vi "Custom SCP Command Page.vi"(8 "error in (no error)":errorcluster, 11 "Node Ptr":T1 format="%.0x") -> (0 "error out":errorcluster)   [LabVIEW 2023, in "Vires VTD System Explorer.lvlib"]
uses:
  Vires VTD System Explorer.lvlib
  <vilib>/NI VeriStand/Custom Device API/Custom Device Item Ref.ctl
  <vilib>/Utility/miscctls.llb/LVRowAndColumnTypeDef.ctl
  Shared/Constants.vi
  <vilib>/NI VeriStand/Custom Device API/Get Item Property (Boolean).vi
  <vilib>/NI VeriStand/Custom Device API/Set Item Property (Boolean).vi
  <vilib>/NI VeriStand/Custom Device API/Custom Device API.lvlib
  Shared/Vires VTD Shared.lvlib
panel:
  in  "Display hidden characters":bool
  in  "Default SCP Command ID":dbl
  in  "Command String":string
  in  "Down Arrow":bool
  in  "Up Arrow":bool
  in  "c SCP List":i32(listbox) caption="Custom SCP Commands List"
  in  "SHDocVw.IWebBrowser2":refnum<k7>(container)
  in  "Header":cluster{"Section Name":string}={"Section Name"="Custom Device Channel Settings"}
  in  "Description":string
  in  "Name":string
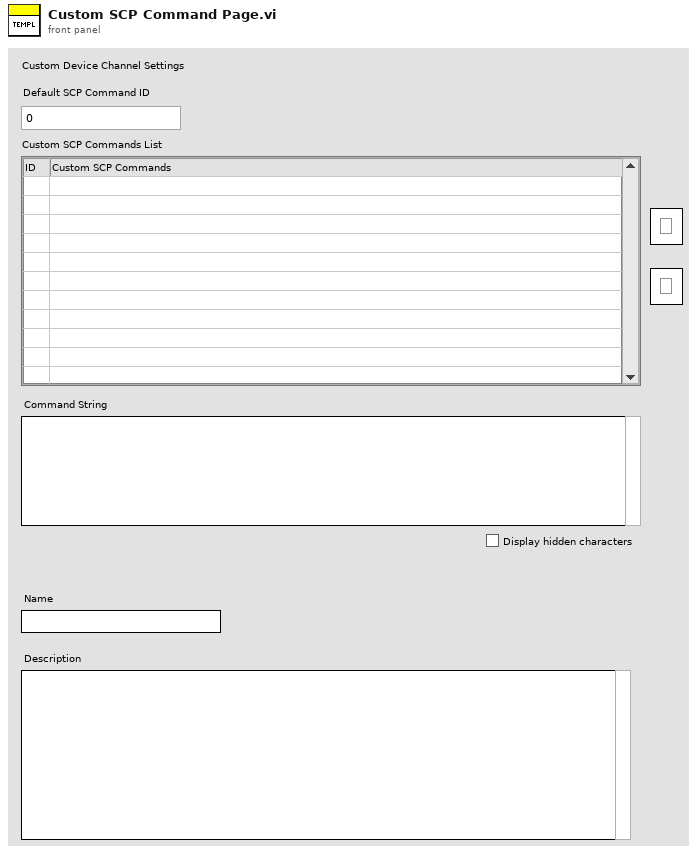
[diagram p1: front panel]
types:
  T1 = typedef "Custom Device API.lvlib/Custom Device Item Ref.ctl" = u64
  T2 = typedef "Custom Device API.lvlib/Custom Device Channel.ctl" = cluster{"Type":T3, "Units":string, "Default Value":dbl, "Faultable":bool, "Scalable":bool}
  T3 = typedef "Custom Device API.lvlib/Custom Device Channel Type.ctl" = enum16{"Input", "Output"}
  T4 = typedef "Custom Device API.lvlib/Custom Device Item Info.ctl" = cluster{"Name":string, "Is Channel":bool, "GUID":string, "Is Waveform":bool}
  T5 = typedef "LVRowAndColumnTypeDef.ctl" = cluster{"Row":i32, "Column":i32}
  T6 = typedef "Custom Device API.lvlib/Custom Device Commands.ctl" = enum16{"Default", "Item renamed", "Shutdown", "Dynamic button pressed"}
  T7 = typedef "LVPoint32TypeDef.ctl" = cluster{"Horizontal":i32, "Vertical":i32}
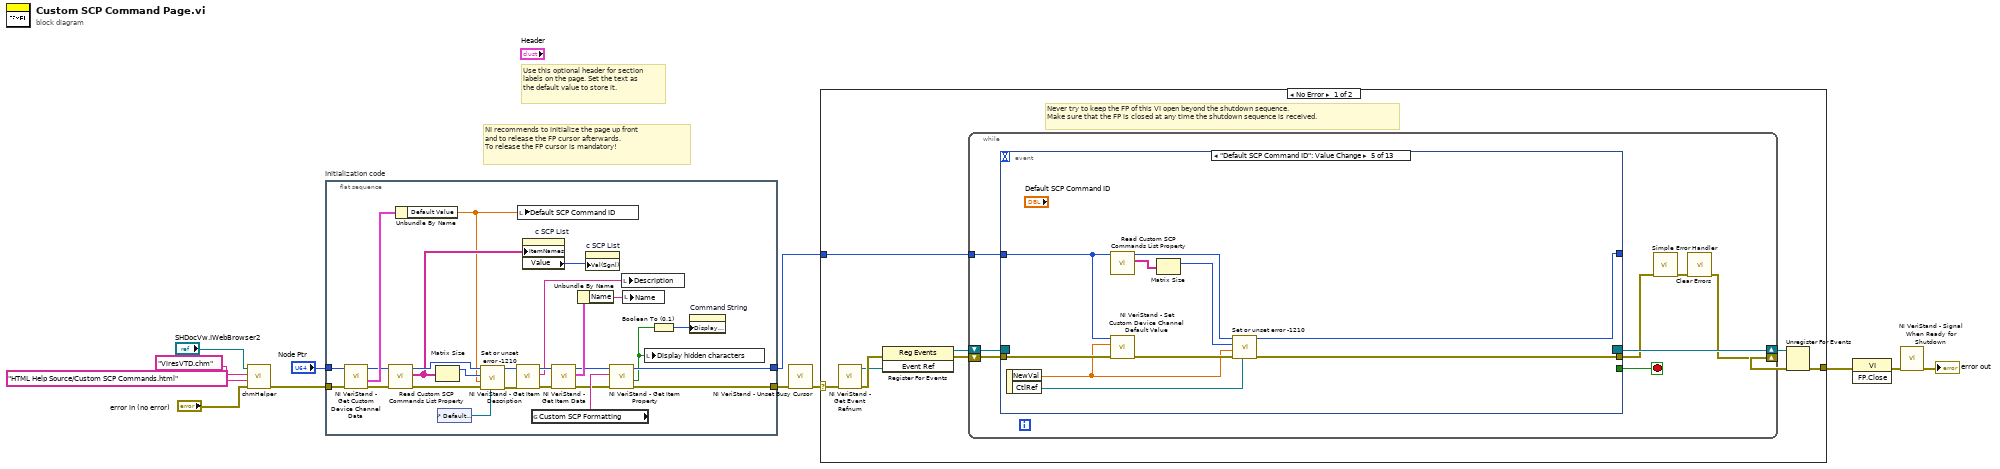
[diagram p0: block diagram]
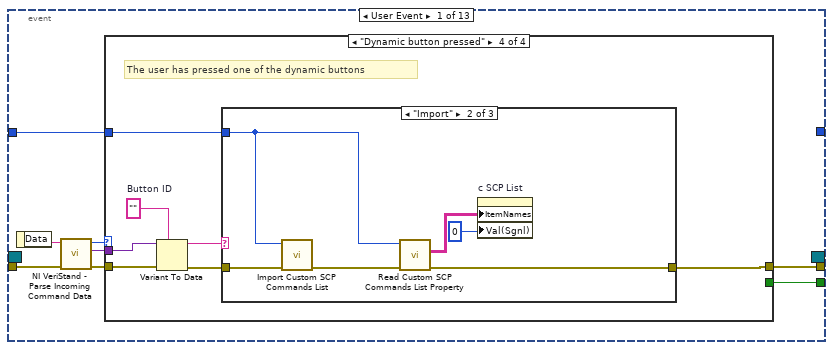
[diagram p2: hidden frame]
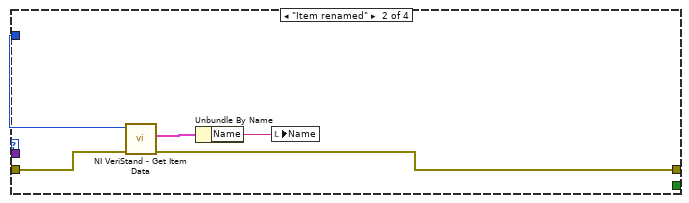
[diagram p4: hidden frame]
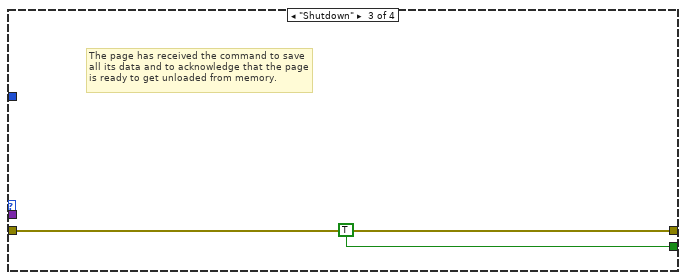
[diagram p5: hidden frame]
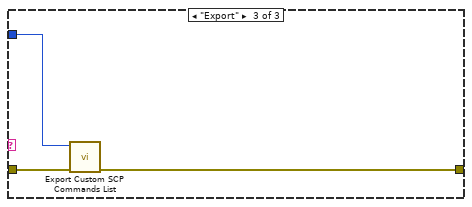
[diagram p7: hidden frame]
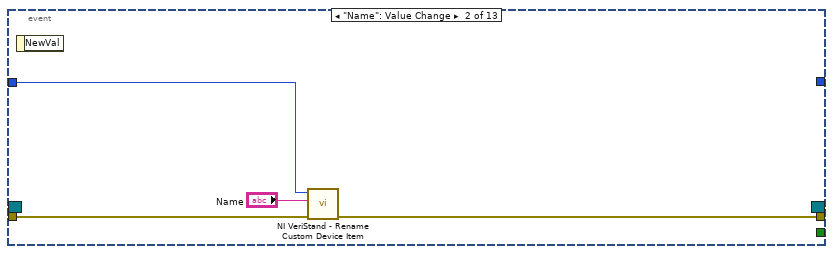
[diagram p8: hidden frame]
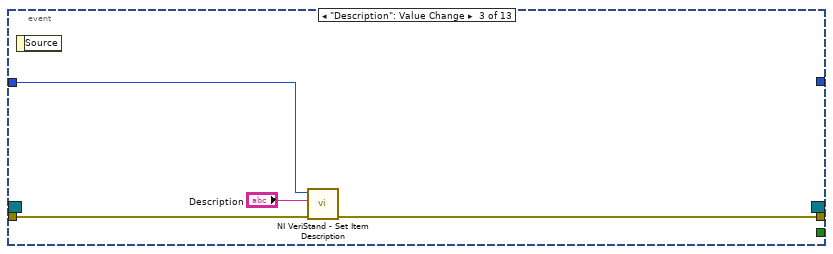
[diagram p9: hidden frame]
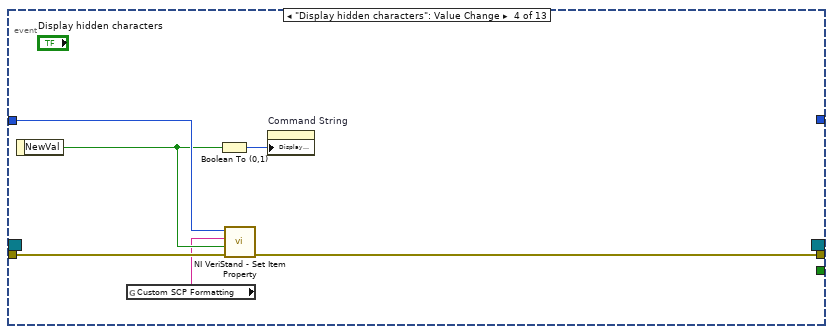
[diagram p10: hidden frame]
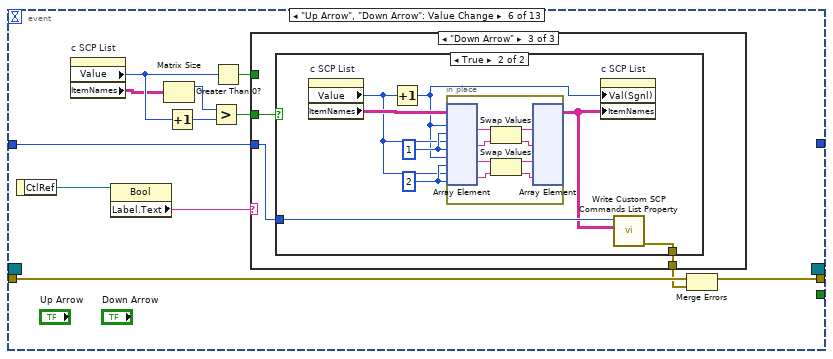
[diagram p11: hidden frame]
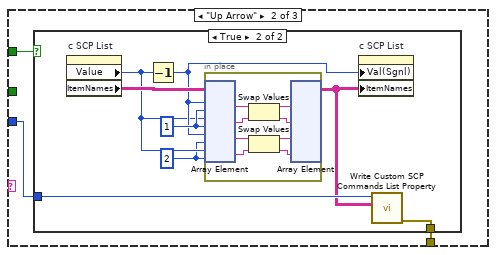
[diagram p13: hidden frame]
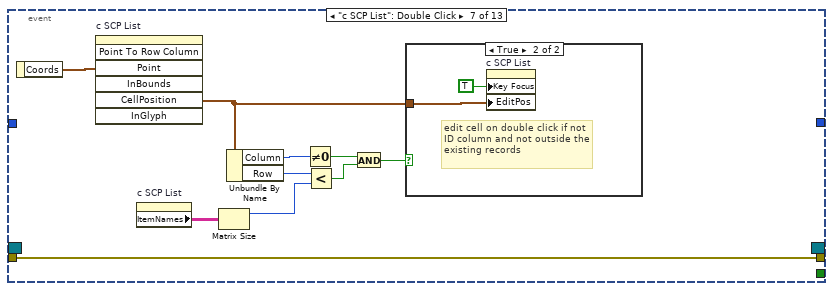
[diagram p16: hidden frame]
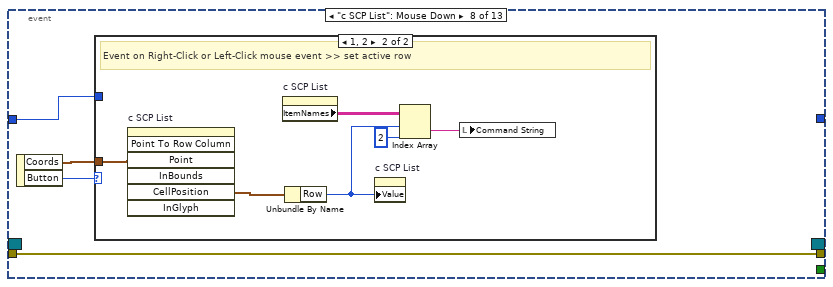
[diagram p18: hidden frame]
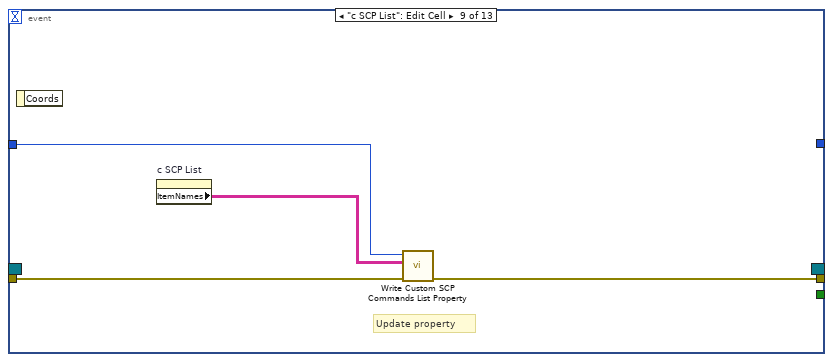
[diagram p20: hidden frame]
diagram:
  # "Use this optional header for section labels on the page. Set the text as the default value to store it."
  # "NI recommends to initialize the page up front\nand to release the FP cursor afterwards.\nTo release the FP cursor is mandatory!"
  n1 = call "chmHelper.vi"("error in (no error)"="error in (no error)", "HTML File"="HTML Help Source/Custom SCP Commands.html", "Main CHM File"="ViresVTD.chm" ("HTML File"), "Automation Refnum in"="SHDocVw.IWebBrowser2") -> ("error out"=w4:errorcluster)  [unwired: 7 in]
  n2 = flat-sequence "Initialization code" {
    tunnel: w4 -> [w29]
    tunnel: "Node Ptr" -> [w33]
    tunnel: [w23] -> w8
    tunnel: [w24] -> w6
    frame #0 {
      n3 = call <vilib>:"NI VeriStand - Get Custom Device Channel Data.vi"("error in (no error)"=w29, "Channel Ref in"=w33) -> ("error out"=w31:errorcluster, "Channel"=w32:T2, "Channel Ref out"=w30:T1)  [unwired: 4 in, 3 out]
      n4 = call "Read Custom SCP Commands List Property.vi"("error in (no error)"=w31, "Node Ptr"=w30) -> ("error out"=w17:errorcluster, "Custom SCP Commands List"=w16:string[][], "Item Ref out"=w18:T1)  [unwired: 7 in]
      n5 = Unbundle By Name(w32) -> ("Default Value"=w13:dbl)
      n6 = Matrix Size(0:w16) -> (1:w20:i32)  [unwired: 1 out]
      n7 = control-ref of="Default SCP Command ID"() -> (w14:refnum<vi>)
      n8 = call "Set or unset error -1210.vi"("ID Control Refnum"=w14, "error in"=w17, "New Default Value"=w13, "# of columns"=w20, "Item Ref In"=w18) -> ("error out"=w15:errorcluster, "Item Ref Out"=w19:T1)  [unwired: 5 in]
      n9 = call <vilib>:"NI VeriStand - Get Item Description.vi"("error in (no error)"=w15, "Item Ref in"=w19) -> ("error out"=w36:errorcluster, "Description"=w37:string, "Item Ref out"=w38:T1)  [unwired: 7 out]
      n10 = local write "Default SCP Command ID"(w13) -> ()
      n11 = property on="c SCP List" class="MCListbox (strict)"("ItemNames"=w16) -> ("Value"=w28:i32)  [unwired: 2 in, 2 out]
      n12 = global read "Constants.vi" "Custom SCP Formatting"() -> (w27:string)
      n13 = call <vilib>:"NI VeriStand - Get Item Data.vi"("error in (no error)"=w36, "Item Ref in"=w38) -> ("error out"=w26:errorcluster, "Item Info"=w35:T4, "Item Ref out"=w25:T1)  [unwired: 7 out]
      n14 = Unbundle By Name(w35) -> ("Name"=w34:string)
      n15 = property on="c SCP List" class="MCListbox (strict)"("Val(Sgnl)"=w28) -> ()  [unwired: 2 in, 2 out]
      n16 = call-poly <vilib>:"NI VeriStand - Get Item Property.vi"("error in (no error)"=w26, "Property Name"=w27, "Item Ref in"=w25) -> ("error out"=w23:errorcluster, "Value"=w21:bool, "Item Ref out"=w24:T1)  [unwired: 5 in, 1 out]
      n17 = local write "Description"(w37) -> ()
      n18 = local write "Name"(w34) -> ()
      n19 = local write "Display hidden characters"(w21) -> ()
      n20 = Boolean To (0,1)(Boolean=w21) -> (0, 1=w22:i16)
      n21 = property on="Command String" class="Str"("Display Style"=w22) -> ()  [unwired: 2 in, 2 out]
    }
  }
  n22 = call <vilib>:"NI VeriStand - Unset Busy Cursor.vi"("error in (no error)"=w8) -> ("error out"=w7:errorcluster)  [unwired: 10 out]
  n23 = case shown="No Error" w7 {
    selector: w7 -> [w39 w260]
    tunnel: [w44 w258] -> w12
    tunnel: w6 -> [w40 _]
    frame No Error {
      # "Never try to keep the FP of this VI open beyond the shutdown sequence.\nMake sure that the FP is closed at any time the shutdown sequence is received."
      n24 = call <vilib>:"NI VeriStand - Get Event Refnum.vi"("error in (no error)"=w39) -> ("error out"=w47:errorcluster, "Event Ref"=w43:refnum<user-event>)  [unwired: 9 out]
      n25 = register-events(error in=w47, w43) -> (reference out=w41:refnum<event-registration>, error out=w42:errorcluster)  [unwired: 1 in]
      n26 = while {
        tunnel: w40 -> [w51]
        shift-right: [w48] -> w45
        shift-left: w42 -> [w54]
        shift-right: [w55] -> w46
        shift-left: w41 -> [w53]
        stop <- w52 stop-if-true
        n27 = event shown="[4] \"Default SCP Command ID\": Value Change" {
          selector: w53 -> [_ _ _ _ _ _ _ _ _ _ _ _ _]
          dyn-events: [_ _ _ _ _ _ _ _ _ _ _ _ _] -> w55
          timeout: _ -> [_ _ _ _ _ _ _ _ _ _ _ _ _]
          tunnel: w54 -> [w63 w92 w95 w101 w110 w123 w168 w177 w186 w196 w202 w208 w211]
          tunnel: [w59 _ _ _ _ _ _ _ _ _ _ _ _] -> w52
          tunnel: [w58 w91 w94 w100 w107 w115 w168 w177 w185 w195 w202 w203 w212] -> w50
          tunnel: w51 -> [w57 w90 w96 w99 w105 w116 _ w175 w187 w197 _ _ w210]
          tunnel: [_ _ _ _ w106 _ _ _ _ _ _ _ _] -> _
          event User Event {
            n28 = event-data() -> ("Data"=w62:string)  [unwired: 1 out]
            n29 = call <vilib>:"NI VeriStand - Parse Incoming Command Data.vi"("error in (no error)"=w63, "Incoming data"=w62) -> ("error out"=w61:errorcluster, "Outgoing data"=w56:variant, "Action"=w60:T6)  [unwired: 7 out]
            n30 = case shown="\"Dynamic button pressed\"" w60 {
              tunnel: w61 -> [w64 w69 w70 w78]
              tunnel: [_ _ TRUE _] -> w59
              tunnel: [w64 w67 w70 w73] -> w58
              tunnel: w57 -> [_ w65 _ w75]
              tunnel: w56 -> [_ _ _ w77]
              frame "Default", Default {
              }
              frame "Item renamed" {
                n31 = call <vilib>:"NI VeriStand - Get Item Data.vi"("error in (no error)"=w69, "Item Ref in"=w65) -> ("error out"=w67:errorcluster, "Item Info"=w68:T4)  [unwired: 8 out]
                n32 = Unbundle By Name(w68) -> ("Name"=w66:string)
                n33 = local write "Name"(w66) -> ()
              }
              frame "Shutdown" {
                # "The page has received the command to save all its data and to acknowledge that the page is ready to get unloaded from memory."
              }
              frame "Dynamic button pressed" {
                w76 = ""  # Button ID
                # "The user has pressed one of the dynamic buttons"
                n34 = Variant To Data(error in=w78, type=w76, Variant=w77) -> (data=w72:string, error out=w74:errorcluster)
                n35 = case shown="\"Import\"" w72 {
                  tunnel: w75 -> [_ w81 w88]
                  tunnel: w74 -> [w79 w85 w87]
                  tunnel: [w79 w82 w86] -> w73
                  frame Default {
                  }
                  frame "Import" {
                    n36 = call "Import Custom SCP Commands List.vi"("error in (no error)"=w85, "Node Ptr"=w81) -> ("error out"=w83:errorcluster)  [unwired: 9 in]
                    n37 = call "Read Custom SCP Commands List Property.vi"("error in (no error)"=w83, "Node Ptr"=w81) -> ("error out"=w82:errorcluster, "Custom SCP Commands List"=w84:string[][])  [unwired: 7 in, 1 out]
                    n38 = property on="c SCP List" class="MCListbox (strict)"("ItemNames"=w84, "Val(Sgnl)"=0 ("Value (Signaling)")) -> ()  [unwired: 2 in, 2 out]
                  }
                  frame "Export" {
                    n39 = call "Export Custom SCP Commands List.vi"("error in (no error)"=w87, "Node Ptr"=w88) -> ("error out"=w86:errorcluster)  [unwired: 9 in]
                  }
                }
              }
            }
          }
          event "Name": Value Change {
            n40 = event-data() -> ()  [unwired: 2 out]
            n41 = call <vilib>:"NI VeriStand - Rename Custom Device Item.vi"("error in (no error)"=w92, "New Name"="Name", "Item Ref in"=w90) -> ("error out"=w91:errorcluster)  [unwired: 1 in, 7 out]
          }
          event "Description": Value Change {
            n42 = event-data() -> ()  [unwired: 2 out]
            n43 = call <vilib>:"NI VeriStand - Set Item Description.vi"("error in (no error)"=w95, "Description"="Description", "Item Ref in"=w96) -> ("error out"=w94:errorcluster)  [unwired: 8 out]
          }
          event "Display hidden characters": Value Change {
            n44 = event-data() -> ("NewVal"=w98:bool)  [unwired: 1 out]
            n45 = global read "Constants.vi" "Custom SCP Formatting"() -> (w97:string)
            n46 = Boolean To (0,1)(Boolean=w98) -> (0, 1=w102:i16)
            n47 = call-poly <vilib>:"NI VeriStand - Set Item Property.vi"("error in (no error)"=w101, "Value"=w98, "Property Name"=w97, "Item Ref in"=w99) -> ("error out"=w100:errorcluster)  [unwired: 5 in, 2 out]
            n48 = property on="Command String" class="Str"("Display Style"=w102) -> ()  [unwired: 2 in, 2 out]
          }
          event "Default SCP Command ID": Value Change {
            n49 = event-data() -> ("NewVal"=w104:dbl, "CtlRef"=w103:refnum<vi>)  [unwired: 1 out]
            n50 = call "Read Custom SCP Commands List Property.vi"("Node Ptr"=w105) -> ("Custom SCP Commands List"=w112:string[][], "Item Ref out"=w108:T1)  [unwired: 8 in, 1 out]
            n51 = call <vilib>:"NI VeriStand - Set Custom Device Channel Default Value.vi"("error in (no error)"=w110, "Default Value"=w104, "Channel Ref in"=w105) -> ("error out"=w109:errorcluster)  [unwired: 7 in, 1 out]
            n52 = Matrix Size(0:w112) -> (1:w111:i32)  [unwired: 1 out]
            n53 = call "Set or unset error -1210.vi"("ID Control Refnum"=w103, "error in"=w109, "New Default Value"=w104, "# of columns"=w111, "Item Ref In"=w108) -> ("error out"=w107:errorcluster, "Item Ref Out"=w106:T1)  [unwired: 5 in]
          }
          event "Up Arrow", "Down Arrow": Value Change {
            n54 = event-data() -> ("CtlRef"=w124:refnum<vi>)  [unwired: 1 out]
            n55 = property on="c SCP List" class="MCListbox (strict)"() -> ("Value"=w121:i32, "ItemNames"=w120:string[][])  [unwired: 2 in, 2 out]
            n56 = property class="Bool"(reference=w124) -> ("Label.Text"=w122:string)  [unwired: 1 in, 2 out]
            n57 = Matrix Size(0:w120) -> (1:w113:i32)  [unwired: 1 out]
            n58 = Increment(x=w121) -> (x+1=w119:i32)
            n59 = Greater?(x=w113, y=w119) -> (0:w118:bool)
            n60 = Greater Than 0?(x=w121) -> (x > 0?=w117:bool)
            n61 = case shown="\"Down Arrow\"" w122 {
              tunnel: w118 -> [_ _ w144]
              tunnel: w117 -> [_ w127 _]
              tunnel: w116 -> [_ w126 w146]
              tunnel: [_ w125 w145] -> w114
              frame Default {
              }
              frame "Up Arrow" {
                n62 = case shown="True" w127 {
                  tunnel: w126 -> [_ w133]
                  tunnel: [_ w132] -> w125
                  frame False {
                  }
                  frame True {
                    w128 = 2
                    w135 = 1
                    n63 = property on="c SCP List" class="MCListbox (strict)"() -> ("Value"=w129:i32, "ItemNames"=w134:string[][])  [unwired: 2 in, 2 out]
                    n64 = Decrement(x=w129) -> (x-1=w130:i32)
                    n65 = in-place {
                      n66 = in-place-array #1(w134, w130, w135, w129, w135, w130, w128, w129, w128) -> (w143:string, w142:string, w139:string, w138:string)
                      n67 = Swap Values(12:w143, 14:w142) -> (1:w141:string, 3:w140:string)  [unwired: 1 out]
                      n68 = Swap Values(12:w139, 14:w138) -> (1:w137:string, 3:w136:string)  [unwired: 1 out]
                      n69 = in-place-array #1(w141, w140, w137, w136) -> (w131:string[][])  [unwired: 8 out]
                    }
                    n70 = property on="c SCP List" class="MCListbox (strict)"("Val(Sgnl)"=w130, "ItemNames"=w131) -> ()  [unwired: 2 in, 2 out]
                    n71 = call "Write Custom SCP Commands List Property.vi"("Custom SCP Commands List"=w131, "Node Ptr"=w133) -> ("error out"=w132:errorcluster)  [unwired: 8 in, 1 out]
                  }
                }
              }
              frame "Down Arrow" {
                n72 = case shown="True" w144 {
                  tunnel: w146 -> [_ w152]
                  tunnel: [_ w151] -> w145
                  frame False {
                  }
                  frame True {
                    w149 = 2
                    w154 = 1
                    n73 = property on="c SCP List" class="MCListbox (strict)"() -> ("Value"=w148:i32, "ItemNames"=w153:string[][])  [unwired: 2 in, 2 out]
                    n74 = Increment(x=w148) -> (x+1=w147:i32)
                    n75 = in-place {
                      n76 = in-place-array #2(w153, w147, w154, w148, w154, w147, w149, w148, w149) -> (w162:string, w161:string, w158:string, w157:string)
                      n77 = Swap Values(12:w162, 14:w161) -> (1:w160:string, 3:w159:string)  [unwired: 1 out]
                      n78 = Swap Values(12:w158, 14:w157) -> (1:w156:string, 3:w155:string)  [unwired: 1 out]
                      n79 = in-place-array #2(w160, w159, w156, w155) -> (w150:string[][])  [unwired: 8 out]
                    }
                    n80 = property on="c SCP List" class="MCListbox (strict)"("Val(Sgnl)"=w147, "ItemNames"=w150) -> ()  [unwired: 2 in, 2 out]
                    n81 = call "Write Custom SCP Commands List Property.vi"("Custom SCP Commands List"=w150, "Node Ptr"=w152) -> ("error out"=w151:errorcluster)  [unwired: 8 in, 1 out]
                  }
                }
              }
            }
            n82 = Merge Errors(w123, w114) -> (w115:errorcluster)
          }
          event "c SCP List": Double Click {
            n83 = event-data() -> ("Coords"=w172:T7)  [unwired: 1 out]
            n84 = invoke on="c SCP List" class="MCListbox (strict)" method="Point To Row Column"("Point"=w172) -> ("CellPosition"=w171:T5)  [unwired: 6 in, 6 out]
            n85 = property on="c SCP List" class="MCListbox (strict)"() -> ("ItemNames"=w164:string[][])  [unwired: 2 in, 2 out]
            n86 = Matrix Size(0:w164) -> (1:w163:i32)  [unwired: 1 out]
            n87 = Unbundle By Name(w171) -> ("Column"=w170:i32, "Row"=w167:i32)
            n88 = Not Equal To 0?(x=w170) -> (x != 0?=w169:bool)
            n89 = Less?(x=w167, y=w163) -> (x < y?=w166:bool)
            n90 = And(x=w169, y=w166) -> (x .and. y?=w165:bool)
            n91 = case shown="True" w165 {
              tunnel: w171 -> [_ w174]
              frame False {
              }
              frame True {
                # "edit cell on double click if not ID column and not outside the existing records"
                n92 = property on="c SCP List" class="MCListbox (strict)"("Key Focus"=TRUE, "EditPos"=w174) -> ()  [unwired: 2 in, 2 out]
              }
            }
          }
          event "c SCP List": Mouse Down {
            n93 = event-data() -> ("Coords"=w178:T7, "Button"=w176:u16)  [unwired: 1 out]
            n94 = case shown="1, 2" w176 {
              tunnel: w178 -> [_ w184]
              tunnel: w175 -> [_ _]
              frame 0, Default {
              }
              frame 1, 2 {
                # "Event on Right-Click or Left-Click mouse event >> set active row"
                n95 = invoke on="c SCP List" class="MCListbox (strict)" method="Point To Row Column"("Point"=w184) -> ("CellPosition"=w183:T5)  [unwired: 6 in, 6 out]
                n96 = property on="c SCP List" class="MCListbox (strict)"() -> ("ItemNames"=w182:string[][])  [unwired: 2 in, 2 out]
                n97 = Unbundle By Name(w183) -> ("Row"=w180:i32)
                n98 = property on="c SCP List" class="MCListbox (strict)"("Value"=w180) -> ()  [unwired: 2 in, 2 out]
                n99 = Index Array(array=w182, index (row)=w180, index (col)=2 ("disabled index (col)")) -> (element=w179:string)
                n100 = local write "Command String"(w179) -> ()
              }
            }
          }
          event "c SCP List": Edit Cell {
            # "Update property"
            n101 = event-data() -> ()  [unwired: 2 out]
            n102 = property on="c SCP List" class="MCListbox (strict)"() -> ("ItemNames"=w188:string[][])  [unwired: 2 in, 2 out]
            n103 = call "Write Custom SCP Commands List Property.vi"("error in (no error)"=w186, "Custom SCP Commands List"=w188, "Node Ptr"=w187) -> ("error out"=w185:errorcluster)  [unwired: 7 in, 1 out]
          }
          event "Command String": Value Change {
            # "Update property"
            n104 = event-data() -> ("NewVal"=w191:string)  [unwired: 1 out]
            n105 = property on="c SCP List" class="MCListbox (strict)"() -> (error out=w194:errorcluster, "ItemNames"=w193:string[][], "Value"=w190:i32)  [unwired: 2 in, 1 out]
            n106 = Replace Array Subset(array=w193, new element=w191, index (row)=w190, index (col)=2 ("disabled index (col)")) -> (w192:string[][])
            n107 = call "Write Custom SCP Commands List Property.vi"("error in (no error)"=w196, "Custom SCP Commands List"=w192, "Node Ptr"=w197) -> ("error out"=w195:errorcluster)  [unwired: 7 in, 1 out]
            n108 = property on="c SCP List" class="MCListbox (strict)"(error in=w194, "ItemNames"=w192) -> ()  [unwired: 1 in, 2 out]
          }
          event "c SCP List": Value Change {
            n109 = event-data() -> ("NewVal"=w198:i32)  [unwired: 1 out]
            n110 = property on="c SCP List" class="MCListbox (strict)"() -> ("ItemNames"=w201:string[][])  [unwired: 2 in, 2 out]
            n111 = Index Array(array=w201, index (row)=w198, index (col)=2 ("disabled index (col)")) -> (element=w199:string)
            n112 = local write "Command String"(w199) -> ()
          }
          event "c SCP List": Shortcut Menu Activation? {
            w204 = string[] ["Add", "Remove", "APP_SEPARATOR", "Remove All"] ("item names")
            n113 = event-data() -> ("Coords"=w207:T7, "MenuRef"=w209:refnum<k9>)  [unwired: 1 out]
            n114 = Delete Menu Items(6:w208, 9:w209) -> (0:w206:errorcluster, 3:w205:refnum<k9>)  [unwired: 2 in]
            n115 = invoke on="c SCP List" class="MCListbox (strict)" method="Point To Row Column"("Point"=w207) -> ()  [unwired: 6 in, 7 out]
            n116 = Insert Menu Items(6:w206, 7:w204, 8:w204, 9:w205) -> (0:w203:errorcluster)  [unwired: 2 in, 2 out]
            n117 = event-data() -> ()  [unwired: 2 in, 1 out]
          }
          event "c SCP List": Shortcut Menu Selection (User) {
            n118 = event-data() -> ("CtlRef"=w215:refnum<vi>, "Coords"=w216:T7, "ItemTag"=w214:string)  [unwired: 1 out]
            n119 = invoke on="Invoke Node" class="MCListbox (strict)" method="Point To Row Column"(reference=w215, "Point"=w216) -> ("CellPosition"=w213:T5)  [unwired: 5 in, 6 out]
            n120 = case shown="\"Remove\"" w214 {
              tunnel: w213 -> [w228 _ _ _]
              tunnel: [w226 w238 w249 w257] -> w212
              tunnel: w211 -> [w225 w237 w249 w257]
              tunnel: w210 -> [w224 w236 _ _]
              frame "Remove" {
                # "Trigger coersion of default ID"
                n121 = Unbundle By Name(w228) -> ("Row"=w227:i32)
                n122 = local write "Command String"("") -> ()
                n123 = property on="c SCP List" class="MCListbox (strict)"() -> ("ItemNames"=w223:string[][])  [unwired: 2 in, 2 out]
                n124 = Delete From Array(array=w223, index (row)=w227) -> (array with subset deleted=w221:string[][])  [unwired: 2 in, 1 out]
                n125 = Delete From Array(array=w221, index (col)=0 ("disabled index (col)")) -> (array with subset deleted=w219:string[][])  [unwired: 2 in, 1 out]
                n126 = for {
                  tunnel: [w230] -> w222 mode=indexing
                  tunnel: w219 -> [w229] mode=indexing
                  i -> [w232]
                  n127 = Format Into String(w232) -> (resulting string=w231:string)  [unwired: 3 in, 1 out]
                  n128 = Build Array (concatenate)(w231, w229) -> (w230:string[])
                }
                n129 = property on="c SCP List" class="MCListbox (strict)"("ItemNames"=w222) -> ()  [unwired: 2 in, 2 out]
                n130 = call "Write Custom SCP Commands List Property.vi"("error in (no error)"=w225, "Custom SCP Commands List"=w222, "Node Ptr"=w224) -> ("error out"=w226:errorcluster)  [unwired: 7 in, 1 out]
                n131 = local read "Default SCP Command ID"() -> (w217:dbl)
                n132 = property on="Default SCP Command ID" class="DigNum (strict)"("Val(Sgnl)"=w217) -> ()  [unwired: 2 in, 2 out]
              }
              frame "Remove All" {
                w235 = string[][] []  # Empty
                # "Trigger coersion of default ID"
                n133 = property on="c SCP List" class="MCListbox (strict)"("ItemNames"=w235) -> ()  [unwired: 2 in, 2 out]
                n134 = call "Write Custom SCP Commands List Property.vi"("error in (no error)"=w237, "Custom SCP Commands List"=w235, "Node Ptr"=w236) -> ("error out"=w238:errorcluster)  [unwired: 7 in, 1 out]
                n135 = property on="Default SCP Command ID" class="DigNum (strict)"("Val(Sgnl)"=0.0 ("Value (Signaling)")) -> ()  [unwired: 2 in, 2 out]
                n136 = local write "Command String"("") -> ()
              }
              frame "Add" {
                w239 = ""
                n137 = property on="c SCP List" class="MCListbox (strict)"() -> ("ItemNames"=w252:string[][])  [unwired: 2 in, 2 out]
                n138 = Delete From Array(array=w252, index (col)=0 ("disabled index (col)")) -> (array with subset deleted=w242:string[][])  [unwired: 2 in, 1 out]
                n139 = Build Array("<Add SCP Command Label>", w239) -> (w240:string[])
                n140 = Build Array (concatenate)(w242, w240) -> (w248:string[][])
                n141 = for {
                  tunnel: [w255] -> w250 mode=indexing
                  tunnel: w248 -> [w254] mode=indexing
                  i -> [w253]
                  n142 = Format Into String(w253) -> (resulting string=w256:string)  [unwired: 3 in, 1 out]
                  n143 = Build Array (concatenate)(w256, w254) -> (w255:string[])
                }
                n144 = local write "Command String"(w239) -> ()
                n145 = Matrix Size(0:w248) -> (1:w247:i32)  [unwired: 1 out]
                n146 = Decrement(x=w247) -> (x-1=w246:i32)
                n147 = Bundle(cluster=T5 {"Row"=0, "Column"=1} ("Edit Position"), "Row"=w246) -> (w245:T5)  [unwired: 1 in]
                n148 = property on="c SCP List" class="MCListbox (strict)"("ItemNames"=w250, "Value"=w246, "Key Focus"=TRUE, "EditPos"=w245) -> ()  [unwired: 2 in, 2 out]
              }
              frame Default {
              }
            }
          }
        }
        n149 = call <vilib>:"Simple Error Handler.vi"("error in (no error)"=w50) -> ("error out"=w49:errorcluster)  [unwired: 1 in, 7 out]
        n150 = call <vilib>:"Clear Errors.vi"("error in (no error)"=w49) -> ("error out"=w48:errorcluster)  [unwired: 1 in, 5 out]
      }
      n151 = Unregister For Events(event registration refnum=w46, error in=w45) -> (error out=w44:errorcluster)
    }
    frame Error {
      n152 = call <vilib>:"Simple Error Handler.vi"("error in (no error)"=w260) -> ("error out"=w259:errorcluster)  [unwired: 1 in, 7 out]
      n153 = call <vilib>:"Clear Errors.vi"("error in (no error)"=w259) -> ("error out"=w258:errorcluster)  [unwired: 1 in, 5 out]
    }
  }
  n154 = invoke class="VI" method="FP.Close"(error in=w12) -> (error out=w11:errorcluster)  [unwired: 2 in, 2 out]
  n155 = call <vilib>:"NI VeriStand - Signal When Ready for Shutdown.vi"("error in (no error)"=w11) -> ("error out"=→"error out":errorcluster)  [unwired: 10 out]
